vi "FTW-Router-Socket Router.vi"(1 "Endpoint":refnum<class "FTW-Endpoint.lvclass">, 2 "Message Handler":refnum<user-event>) -> ()   [LabVIEW 2013, in "FTW-Router.lvclass"]
uses:
  FTW-Router.lvclass
  Message/Request/FTW-Message-IncomingRequest.lvclass
  Endpoint/FTW-Endpoint.lvclass
panel:
  out "Messages Handled":u32
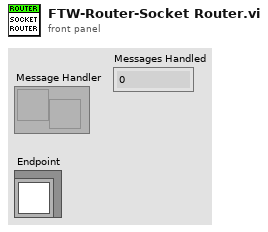
[diagram p1: front panel]
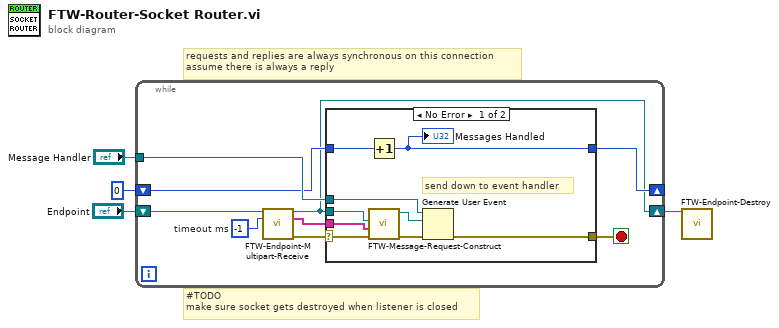
[diagram p0: block diagram]
diagram:
  # "#TODO\nmake sure socket gets destroyed when listener is closed"
  # "requests and replies are always synchronous on this connection\nassume there is always a reply"
  n1 = while {
    tunnel: "Message Handler" -> [w13]
    shift-right: [w5] -> w2
    shift-left: "Endpoint" -> [w12]
    shift-right: [w6] -> _
    shift-left: u32 0 -> [w7]
    stop <- w8 stop-if-true
    w11 = -1  # timeout ms
    n2 = call-dynamic "FTW-Endpoint-Multipart-Receive.vi"("FTW Endpoint"=w12, "Timeout"=w11) -> ("FTW Endpoint out"=w5:refnum<class "FTW-Endpoint.lvclass">, "Message Received"=w9:string[], "error out"=w10:errorcluster)  [unwired: 10 in, 1 out]
    n3 = case shown="No Error" w10 {
      selector: w10 -> [w19 w24]
      tunnel: w13 -> [w22 _]
      tunnel: w9 -> [w14 _]
      tunnel: [w16 w24] -> w8
      tunnel: w5 -> [w15 _]
      tunnel: w7 -> [w21 w23]
      tunnel: [w20 w23] -> w6
      frame No Error {
        # "send down to event handler"
        n4 = Increment(x=w21) -> (x+1=w20:u32)
        "Messages Handled" <- w20
        n5 = call "FTW-Message-Request-Construct.vi"("error in"=w19, "Multipart Message"=w14, "Frontend Endpoint"=w15) -> ("error out"=w18:errorcluster, "FTW Incoming Request"=w17:refnum<class "FTW-Message-IncomingRequest.lvclass">)  [unwired: 7 in]
        n6 = Generate User Event(user event=w22, event data cluster=w17, error in=w18) -> (error out=w16:errorcluster)  [unwired: 1 in, 1 out]
      }
      frame Error {
      }
    }
  }
  n7 = call-dynamic "FTW-Endpoint-Destroy.vi"("FTW Endpoint"=w2) -> ()  [unwired: 14 in, 1 out]
